vi "局部变量.vi"() -> ()   [LabVIEW 2023]
panel:
  out "例子二下":i32
  out "例子二上":i32
  out "例子一 上":i32
  out "例子一下":i32
  in  "例子二":bool
  in  "例子一":bool
  out "concatenated string":string
  out "s? t:f":string
  in  "String":string
  # "局部变量"
  # "Consider the local var is a memory block for the VI.  这个本地变量，不需要和其  VI  连线\n和其  VI  共享 内存 （无论其控件是输入还是输出）"
  # "只有例子1 才能控制两个不同线程 同时 停止。"
  # "多线程控制的时候 ， 会使用到 局部变量， 如这个例子一， 不可以\n把控制变量 （boolean  ）连到 循环外来控制 因为 只有在循环结束以后，\n才会把变量传到循环外边如例子二。"
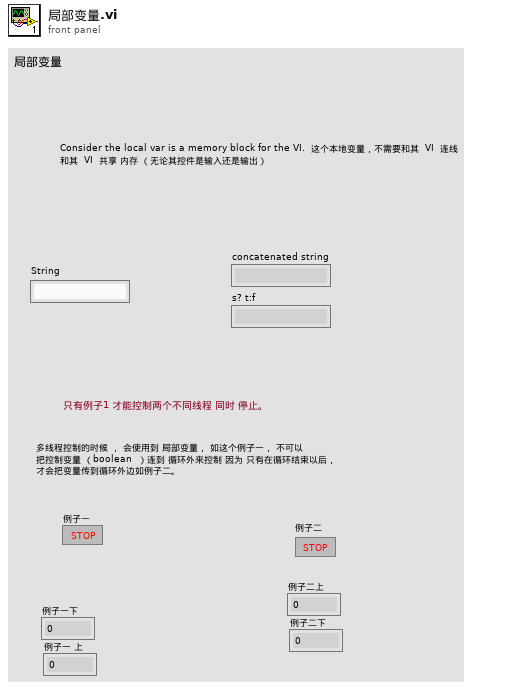
[diagram p1: front panel]
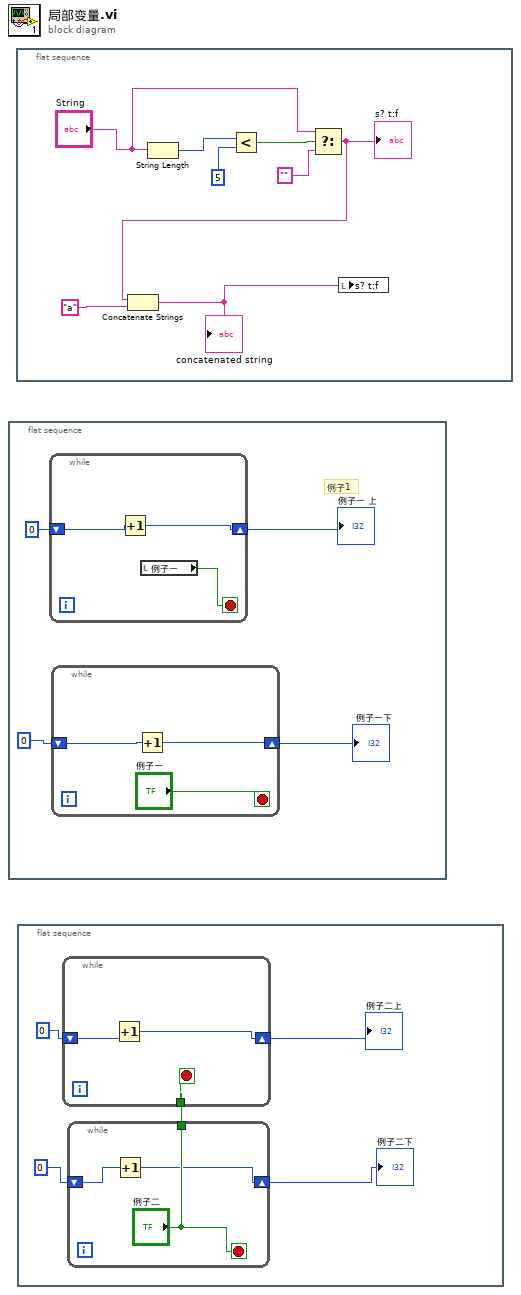
[diagram p0: block diagram]
diagram:
  n1 = flat-sequence {
    frame #0 {
      # "例子1"
      n2 = while {
        shift-right: [w8] -> w2
        shift-left: 0 -> [w10]
        stop <- w9 stop-if-true
        n3 = Increment(x=w10) -> (x+1=w8:i32)
        n4 = local read "例子一"() -> (w9:bool)
      }
      "例子一 上" <- w2
      n5 = while {
        shift-right: [w5] -> w1
        shift-left: 0 -> [w7]
        stop <- "例子一" stop-if-true
        n6 = Increment(x=w7) -> (x+1=w5:i32)
      }
      "例子一下" <- w1
    }
  }
  n7 = flat-sequence {
    frame #0 {
      n8 = String Length(string="String") -> (length=w18:i32)
      n9 = Less?(x=w18, y=5) -> (x < y?=w16:bool)
      n10 = Select(t="String", s=w16, f="") -> (s? t:f=w13:string)
      "s? t:f" <- w13
      n11 = Concatenate Strings(w13, "a") -> (w12:string)
      "concatenated string" <- w12
      n12 = local write "s? t:f"(w12) -> ()
    }
  }
  n13 = flat-sequence {
    frame #0 {
      n14 = while {
        tunnel: ["例子二"] -> w21
        shift-right: [w24] -> w19
        shift-left: 0 -> [w26]
        stop <- "例子二" stop-if-true
        n15 = Increment(x=w26) -> (x+1=w24:i32)
      }
      "例子二下" <- w19
      n16 = while {
        tunnel: w21 -> [w28]
        shift-right: [w27] -> w20
        shift-left: 0 -> [w29]
        stop <- w28 stop-if-true
        n17 = Increment(x=w29) -> (x+1=w27:i32)
      }
      "例子二上" <- w20
    }
  }
